vi "ToggleValve.vi"(0 "object in":refnum<class "CetoniPump.lvclass">, 2 "ValveControl":cluster{"index":i32, "Valve Position":bool}, 5 "error in (no error)":errorcluster) -> (14 "object out":refnum<class "CetoniPump.lvclass">, 19 "error out":errorcluster)   [LabVIEW 2021, in "CetoniPump.lvclass"]
uses:
  CetoniPump.lvclass
  CetoniPump.lvclass/CetoniPump.ctl
  CETONI_SDK/lib/labview/labbCAN_Valve_API/labbCAN_Valve_API.lvlib
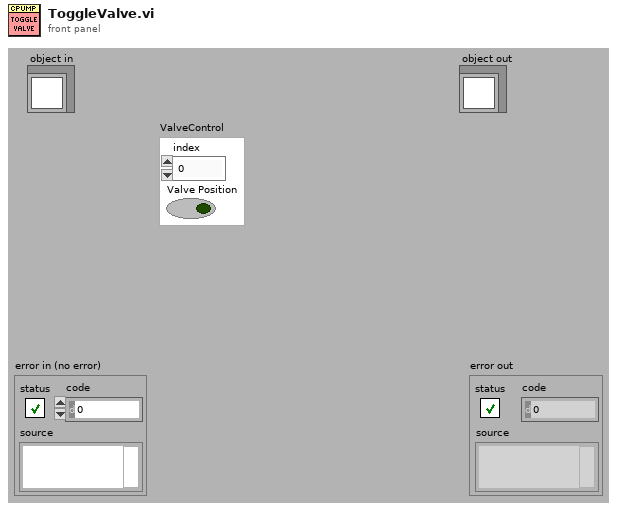
[diagram p1: front panel]
types:
  T1 = cluster{"Pump Handle":i64, "Pump Name":string, "Maximum Volume":dbl, "Maximum Flow Rate":dbl, "Flow Rate":dbl, "Target Level":dbl, "Valve Handle":i64, "Has Valve?":bool, "Actual valve position":i32}[]
  T2 = cluster{"Pump Handle":i64, "Pump Name":string, "Maximum Volume":dbl, "Maximum Flow Rate":dbl, "Flow Rate":dbl, "Target Level":dbl, "Valve Handle":i64, "Has Valve?":bool, "Actual valve position":i32}
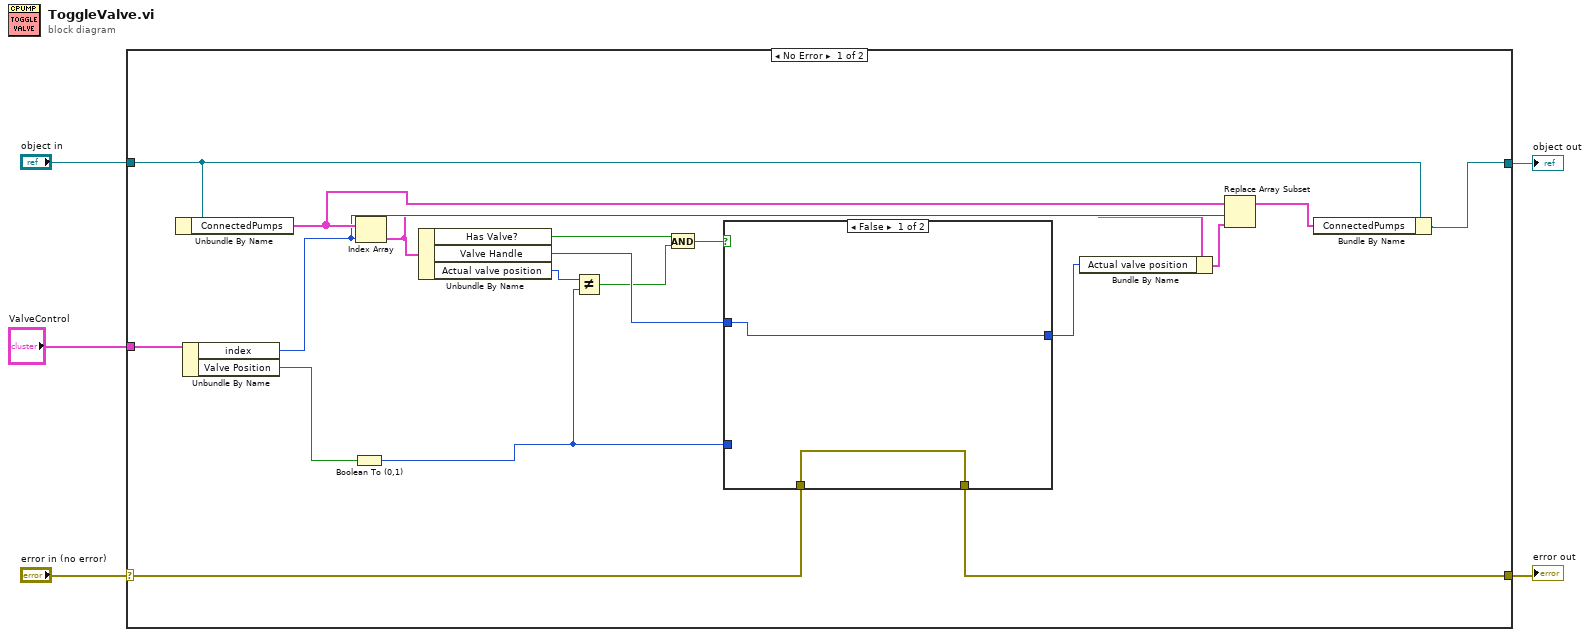
[diagram p0: block diagram]
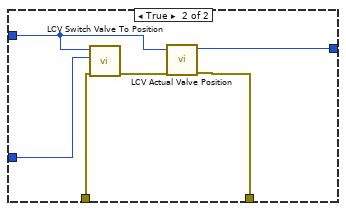
[diagram p2: hidden frame]
diagram:
  n1 = case shown="No Error" "error in (no error)" {
    selector: "error in (no error)" -> [w23 w33]
    tunnel: [w22 w33] -> w4
    tunnel: [w17 w32] -> w2
    tunnel: "object in" -> [w16 w32]
    tunnel: "ValveControl" -> [w19 _]
    frame No Error {
      n2 = Unbundle By Name(w16) -> ("ConnectedPumps"=w15:T1)
      n3 = Unbundle By Name(w19) -> ("index"=w14:i32, "Valve Position"=w18:bool)
      n4 = Boolean To (0,1)(Boolean=w18) -> (0, 1=w8:i16)
      n5 = Index Array(array=w15, index=w14) -> (element=w13:T2)
      n6 = Unbundle By Name(w13) -> ("Has Valve?"=w21:bool, "Valve Handle"=w20:i64, "Actual valve position"=w9:i32)
      n7 = Not Equal?(x=w9, y=w8) -> (x != y?=w6:bool)
      n8 = And(x=w21, y=w6) -> (x .and. y?=w7:bool)
      n9 = case shown="False" w7 {
        tunnel: w8 -> [_ w31]
        tunnel: w23 -> [w25 w30]
        tunnel: [w25 w29] -> w22
        tunnel: w20 -> [w24 w27]
        tunnel: [w24 w26] -> w11
        frame False {
        }
        frame True {
          n10 = call "LCV Switch Valve To Position.vi"("error in (no error)"=w30, "Logical Valve Position"=w31, "Valve Handle"=w27) -> ("error out"=w28:errorcluster)  [unwired: 8 in]
          n11 = call "LCV Actual Valve Position.vi"("error in (no error)"=w28, "Valve Handle"=w27) -> ("error out"=w29:errorcluster, "Actual valve position"=w26:i32)  [unwired: 8 in]
        }
      }
      n12 = Bundle By Name(cluster=w13, "Actual valve position"=w11) -> (w12:T2)
      n13 = Replace Array Subset(array=w15, new element=w12, index=w14) -> (w10:T1)
      n14 = Bundle By Name(cluster=w16, "ConnectedPumps"=w10) -> (w17:refnum<class "CetoniPump.lvclass">)
    }
    frame Error {
    }
  }
  "error out" <- w4
  "object out" <- w2
